vi "Get Ports Section.vi"(8 "error in":errorcluster, 11 "custom device ref":T1 format="%.0x") -> (0 "error out":errorcluster, 1 "All Ports Refs":T1[](array[typedef]) format="%.0x", 2 "Ports Page Ref":T1 format="%.0x", 3 "custom device ref out":T1 format="%.0x")   [LabVIEW 2020, in "AIM ARINC 664 Scripting.lvlib"]
uses:
  AIM ARINC 664 Scripting.lvlib
  <vilib>/NI VeriStand/Custom Device API/Custom Device Item Ref.ctl
  Constants.vi
  <vilib>/NI VeriStand/Custom Device Tools/Custom Device Utility Library/NI VeriStand - Search for Item by GUID.vi
  <vilib>/NI VeriStand/Custom Device Tools/Custom Device Utility Library/Custom Device Utility Library.lvlib
  <vilib>/NI VeriStand/Custom Device Tools/Custom Device Utility Library/NI VeriStand - Search for All Items by GUID.vi
  <vilib>/NI VeriStand/Custom Device API/Custom Device API.lvlib
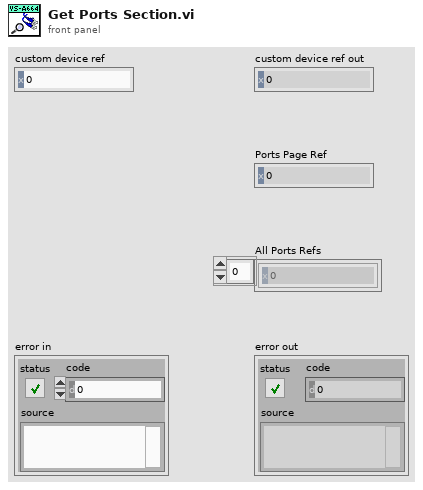
[diagram p1: front panel]
types:
  T1 = typedef "Custom Device API.lvlib/Custom Device Item Ref.ctl" = u64
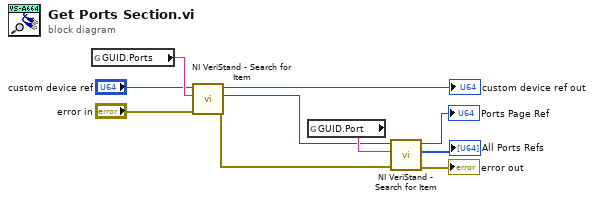
[diagram p0: block diagram]
diagram:
  n1 = global read "Constants.vi" "GUID.Ports"() -> (w8:string)
  n2 = call-poly <vilib>:"NI VeriStand - Search for Item.vi"("error in"="error in", "Item GUID"=w8, "Section Ref in"="custom device ref") -> ("error out"=w2:errorcluster, "Item Ref"=w5:T1, "Section Ref out"=→"custom device ref out":T1)  [unwired: 5 in, 1 out]
  n3 = global read "Constants.vi" "GUID.Port"() -> (w6:string)
  n4 = call-poly <vilib>:"NI VeriStand - Search for Item.vi"("error in"=w2, "Item GUID"=w6, "Section Ref in"=w5) -> ("error out"=→"error out":errorcluster, "Item Refs"=→"All Ports Refs":T1[], "Section Ref out"=→"Ports Page Ref":T1)  [unwired: 5 in, 1 out]
